vi "totalTime.vi"(0 "Rooms":i32(slide) scale=1.0..8.0, 1 "Do You Want To Clean The LivingRoom?":bool, 2 "Return To Home Position":bool, 3 "X":dbl min=-200.0 max=200.0 step=1.0, 4 "Y":dbl min=-200.0 max=200.0 step=1.0) -> (5 "Total Time:":i32)   [LabVIEW 2013]
uses:
  Global 1.vi
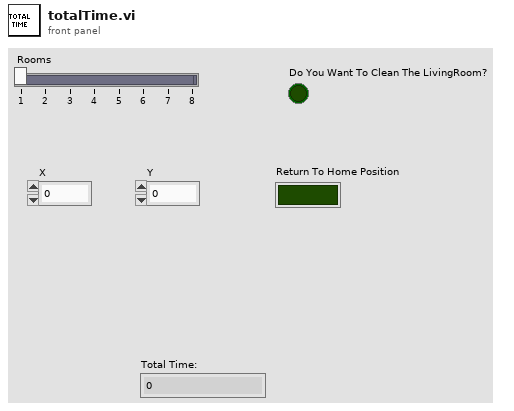
[diagram p1: front panel]
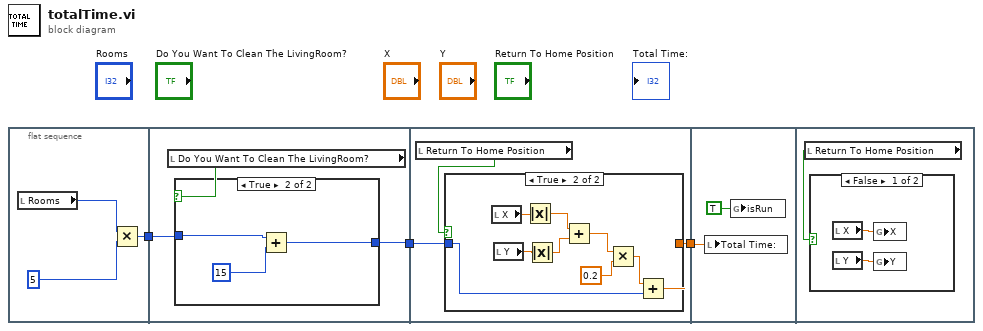
[diagram p0: block diagram]
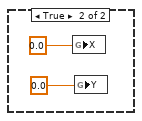
[diagram p4: hidden frame]
diagram:
  n1 = flat-sequence {
    tunnel: [w4] -> w3
    tunnel: w3 -> [w8]
    tunnel: [w9] -> w2
    tunnel: w2 -> [w15]
    tunnel: [w14] -> w1
    tunnel: w1 -> [w28]
    frame #0 {
      n2 = local read "Rooms"() -> (w5:i32)
      n3 = Multiply(x=w5, y=5) -> (x*y=w4:i32)
    }
    frame #1 {
      n4 = local read "Do You Want To Clean The LivingRoom?"() -> (w7:bool)
      n5 = case shown="True" w7 {
        tunnel: [w10 w12] -> w9
        tunnel: w8 -> [w10 w11]
        frame False {
        }
        frame True {
          n6 = Add(x=w11, y=15) -> (x+y=w12:i32)
        }
      }
    }
    frame #2 {
      n7 = local read "Return To Home Position"() -> (w16:bool)
      n8 = case shown="True" w16 {
        tunnel: w15 -> [w17 w19]
        tunnel: [w17 w18] -> w14
        frame False {
        }
        frame True {
          n9 = local read "X"() -> (w25:dbl)
          n10 = local read "Y"() -> (w26:dbl)
          n11 = Absolute Value(x=w25) -> (abs(x)=w23:dbl)
          n12 = Absolute Value(x=w26) -> (abs(x)=w24:dbl)
          n13 = Add(x=w23, y=w24) -> (x+y=w22:dbl)
          n14 = Multiply(x=w22, y=0.2) -> (x*y=w20:dbl)
          n15 = Add(x=w20, y=w19) -> (x+y=w18:dbl)
        }
      }
    }
    frame #3 {
      n16 = local write "Total Time:"(w28) -> ()
      n17 = global write "Global 1.vi" "isRun"(TRUE ("isRun")) -> ()
    }
    frame #4 {
      n18 = local read "Return To Home Position"() -> (w29:bool)
      n19 = case shown="False" w29 {
        frame False {
          n20 = local read "X"() -> (w31:dbl)
          n21 = local read "Y"() -> (w30:dbl)
          n22 = global write "Global 1.vi" "X"(w31) -> ()
          n23 = global write "Global 1.vi" "Y"(w30) -> ()
        }
        frame True {
          n24 = global write "Global 1.vi" "X"(0.0) -> ()
          n25 = global write "Global 1.vi" "Y"(0.0) -> ()
        }
      }
    }
  }
